vi "Konwersja współrzędnej na stopnie dziesiętne.vi"(0 "Kierunek":string, 2 "D":ext, 3 "M":ext, 5 "S":ext format="%.10g") -> (7 "Współrzędna dziesiętna":ext format="%.20g")   [LabVIEW 2015, in "Biblioteka moduł map v3.lvlib" / "Konwersja wsp.lvlib"]
doc: "Zadaniem pliku jest przeliczenie współrzędnej do postaci dziesiętnej z uwzględnieniem kierunku geograficznego. Dla NE wartość współrzędnej przyjmowana jest jako dodadtnia, a dla WS jako ujemna. Do przeliczenia wymagane jest podanie kierunku oraz współrzędnej w stopniach. Minuty i sekundy są opcjonalne. Plik umożliwia przeliczanie współrzędnej podanej w postaci D, DM, DMS wraz z kierunkiem na odpowiednią liczbę dziesiętną."
uses:
  Konwersja wsp.lvlib
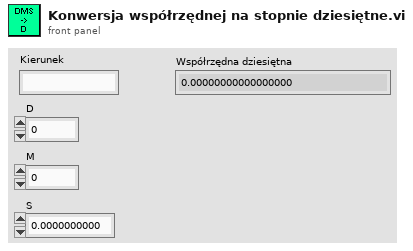
[diagram p1: front panel]
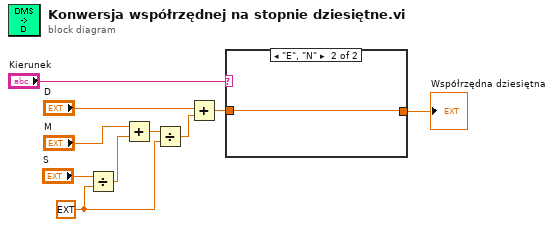
[diagram p0: block diagram]
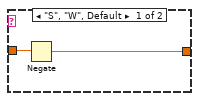
[diagram p2: hidden frame]
diagram:
  w1 = ext 60.0 ("y")
  n1 = Divide(x="S", y=w1) -> (x/y=w9:ext)
  n2 = Add(x="M", y=w9) -> (x+y=w8:ext)
  n3 = Divide(x=w8, y=w1) -> (x/y=w7:ext)
  n4 = Add(x="D", y=w7) -> (x+y=w4:ext)
  n5 = case shown="\"E\", \"N\"" "Kierunek" {
    tunnel: w4 -> [w12 w13]
    tunnel: [w11 w13] -> w3
    frame "S", "W", Default {
      n6 = Negate(x=w12) -> (-x=w11:ext)
    }
    frame "E", "N" {
    }
  }
  "Współrzędna dziesiętna" <- w3
